vi "get http file.vi"(8 "error in (no error)":errorcluster caption="错误输入（无错误）", 10 "timeout (10000)":i32=300000, 11 "http client 输入":refnum<class "http client.lvclass">) -> (0 "error out":errorcluster caption="错误输出", 2 "appended path":path, 3 "http client 输出":refnum<class "http client.lvclass">)   [LabVIEW 2016, in "数据传输系统.lvlib" / "update.lvlib" / "http client.lvclass"]
uses:
  http client.lvclass
  http client.lvclass/http client.ctl
  <vilib>/httpClient/LabVIEWHTTPClient.lvlib
  update.lvlib
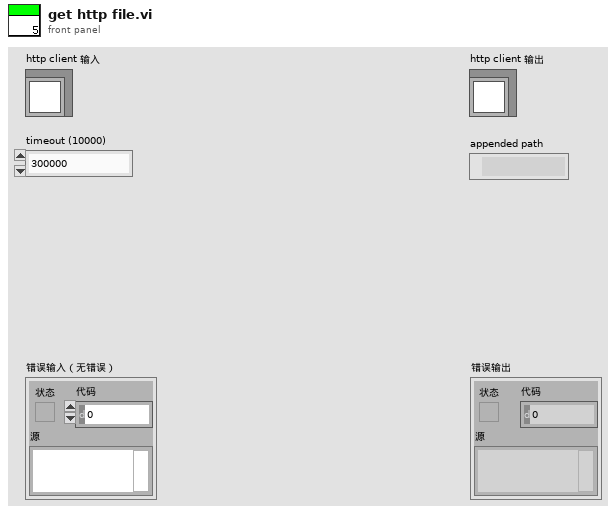
[diagram p1: front panel]
types:
  T1 = typedef "LabVIEWHTTPClient.lvlib/ClientHandle.ctl" = refnum<k1>
  T2 = cluster{"host":string, "port":u16, "user":string, "password":string}
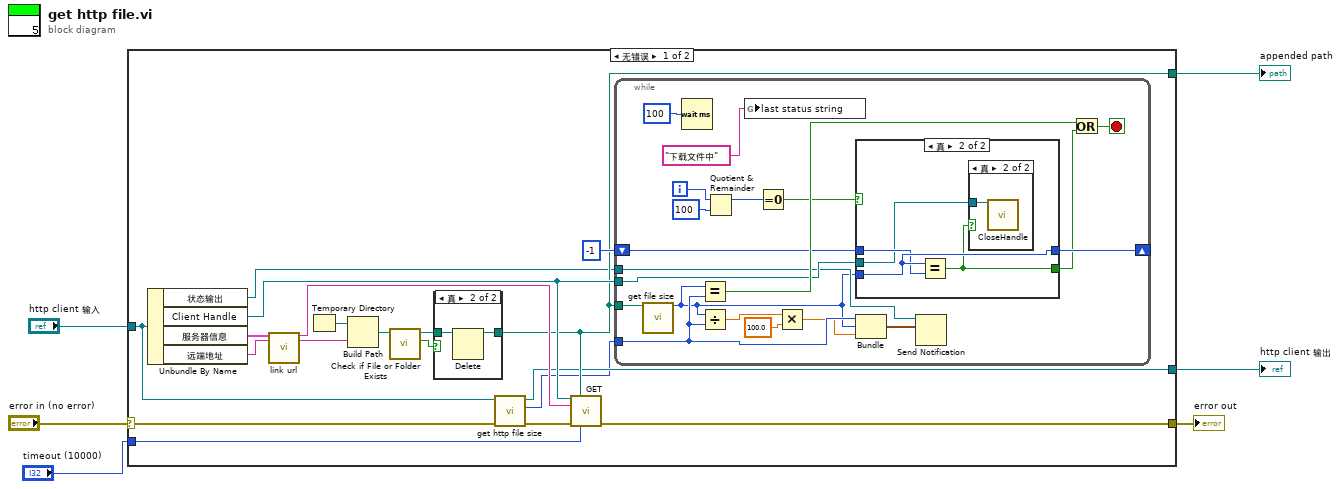
[diagram p0: block diagram]
diagram:
  n1 = case shown="无错误" "error in (no error)" {
    selector: "error in (no error)" -> [w11 w56]
    tunnel: [w21 w56] -> w5
    tunnel: [w12 w55] -> w3
    tunnel: "http client 输入" -> [w13 w55]
    tunnel: [w15 _] -> w2
    tunnel: "timeout (10000)" -> [w7 _]
    frame No Error {
      n2 = Unbundle By Name(w13) -> ("状态输出"=w8:refnum<notifier>, "Client Handle"=w18:T1, "服务器信息"=w25:T2, "远端地址"=w24:string)
      n3 = call "link url.vi"("服务器信息"=w25, "远端地址"=w24) -> ("url"=w20:string, "file name"=w22:string)  [unwired: 16 in]
      n4 = Temporary Directory() -> (w23:path)
      n5 = Build Path(base path=w23, name or relative path=w22) -> (appended path=w17:path)
      n6 = call <vilib>:"Check if File or Folder Exists.vi"("path"=w17) -> ("file or folder exists?"=w14:bool, "dup path"=w16:path)  [unwired: 8 in, 1 out]
      n7 = case shown="真" w14 {
        tunnel: w16 -> [w26 w28]
        tunnel: [w26 w27] -> w15
        frame False {
        }
        frame True {
          n8 = Delete(path (use dialog)=w28) -> (deleted path=w27:path)  [unwired: 4 in, 2 out]
        }
      }
      n9 = call "get http file size.vi"("error in (no error)"=w11, "http client 输入"=w13) -> ("error out"=w10:errorcluster, "文件大小"=w9:i64, "http client 输出"=w12:refnum<class "http client.lvclass">)  [unwired: 7 in]
      n10 = call <vilib>:"GET.vi"("client handle"=w18, "output file"=w15, "url"=w20, "error in (no error)"=w10, "timeout (10000)"=w7) -> ("error out"=w21:errorcluster)  [unwired: 7 in, 3 out]
      n11 = while {
        tunnel: w15 -> [w48]
        shift-right: [w39] -> _
        shift-left: i64 -1 ("size (in bytes)") -> [w38]
        tunnel: w18 -> [w35]
        tunnel: w9 -> [w33]
        tunnel: w8 -> [w34]
        i -> [w42]
        stop <- w44 stop-if-true
        n12 = call "get file size.vi"("file path"=w48) -> ("size (in bytes)"=w32:i64)  [unwired: 18 in]
        n13 = Wait (ms)(milliseconds to wait=u32 100 ("等待时间（毫秒）")) -> ()  [unwired: 1 out]
        n14 = Equal?(x=w32, y=w33) -> (x = y?=w45:bool)
        n15 = Divide(x=w32, y=w33) -> (x/y=w46:dbl)
        n16 = Quotient & Remainder(x=w42, y=100) -> (x-y*floor(x/y)=w40:i32)  [unwired: 1 out]
        n17 = global write "更新全局变量.vi" "last status string"("下载文件中" ("last status string")) -> ()
        n18 = Equal To 0?(x=w40) -> (x = 0?=w37:bool)
        n19 = Multiply(x=w46, y=100.0) -> (x*y=w31:dbl)
        n20 = case shown="真" w37 {
          tunnel: w32 -> [_ w53]
          tunnel: [w49 w53] -> w39
          tunnel: w38 -> [w49 w52]
          tunnel: [_ w51] -> w36
          tunnel: w35 -> [_ w50]
          frame False {
          }
          frame True {
            n21 = Equal?(x=w53, y=w52) -> (x = y?=w51:bool)
            n22 = case shown="真" w51 {
              tunnel: w50 -> [_ w54]
              frame False {
              }
              frame True {
                n23 = call <vilib>:"CloseHandle.vi"("client handle"=w54) -> ()  [unwired: 14 in, 1 out]
              }
            }
          }
        }
        n24 = Bundle("文件大小"=w33, "size (in bytes)"=w32, w31) -> (w30:cluster{"文件大小":i64, "size (in bytes)":i64, dbl})  [unwired: 1 in]
        n25 = Send Notification(notification=w30, notifier=w34) -> ()  [unwired: 1 in, 2 out]
        n26 = Or(x=w45, y=w36) -> (x .or. y?=w44:bool)
      }
    }
    frame Error {
    }
  }
  "error out" <- w5
  "http client 输出" <- w3
  "appended path" <- w2
